vi "Post-Install Custom Action.vi"() -> (0 "error out":errorcluster)   [LabVIEW 2014]
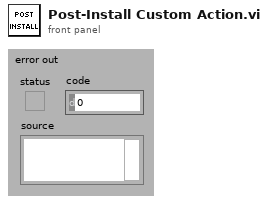
[diagram p1: front panel]
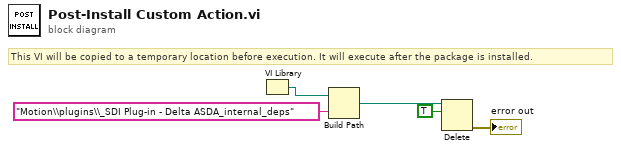
[diagram p0: block diagram]
diagram:
  # "This VI will be copied to a temporary location before execution. It will execute after the package is installed."
  n1 = VI Library() -> (path=w5:path)
  n2 = Build Path(base path=w5, name or relative path="Motion\\plugins\\_SDI Plug-in - Delta ASDA_internal_deps") -> (appended path=w3:path)
  n3 = Delete(path (use dialog)=w3, entire hierarchy (F)=TRUE) -> (error out=→"error out":errorcluster)  [unwired: 3 in, 2 out]
